vi "Get Descriptor_Mod.vi"(0 "VISA resource name":refnum<visa-resource-name>, 5 "Source (0: Channel 1)":u16(ring) items=["Channel 1", "Channel 2", "Channel 3", "Channel 4", "Memory 1", "Memory 2", "Memory 3", "Memory 4", "Function 1", "Function 2", "Function 3", "Function 4", "Function 5", "Function 6", "Function 7", "Function 8", "Other"], 7 "Custom Source ID":string, 11 "error in (no error)":errorcluster) -> (1 "First Valid Point":i32, 2 "Last Valid Point":i32, 3 "Horizontal interval":sgl, 4 "VISA resource name out":refnum<visa-resource-name>, 6 "Vertical gain":sgl, 8 "Horizontal Offset":dbl, 10 "Vertical offset":sgl, 12 "Number Of Data Points":i32, 13 "Nom_Bits":i16, 14 "Command type":i16, 15 "error out":errorcluster)   [LabVIEW 2022 SP3]
doc: "Get basic information about acquisition waveform from specified channel."
uses:
  <instrlib>/LeCroy Wave Series/LeCroy Wave Series.lvlib
panel:
  out "Trigger Time":T1
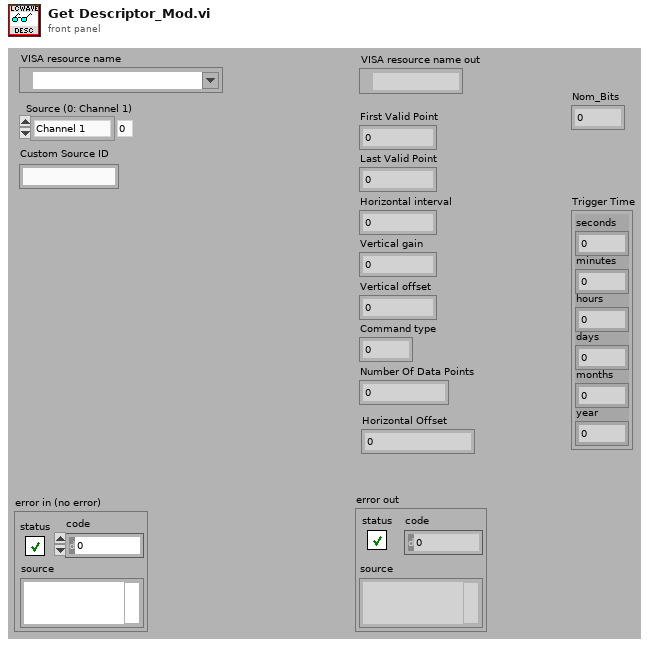
[diagram p1: front panel]
types:
  T1 = cluster{"seconds":dbl, "minutes":u8, "hours":u8, "days":u8, "months":u8, "year":u16}
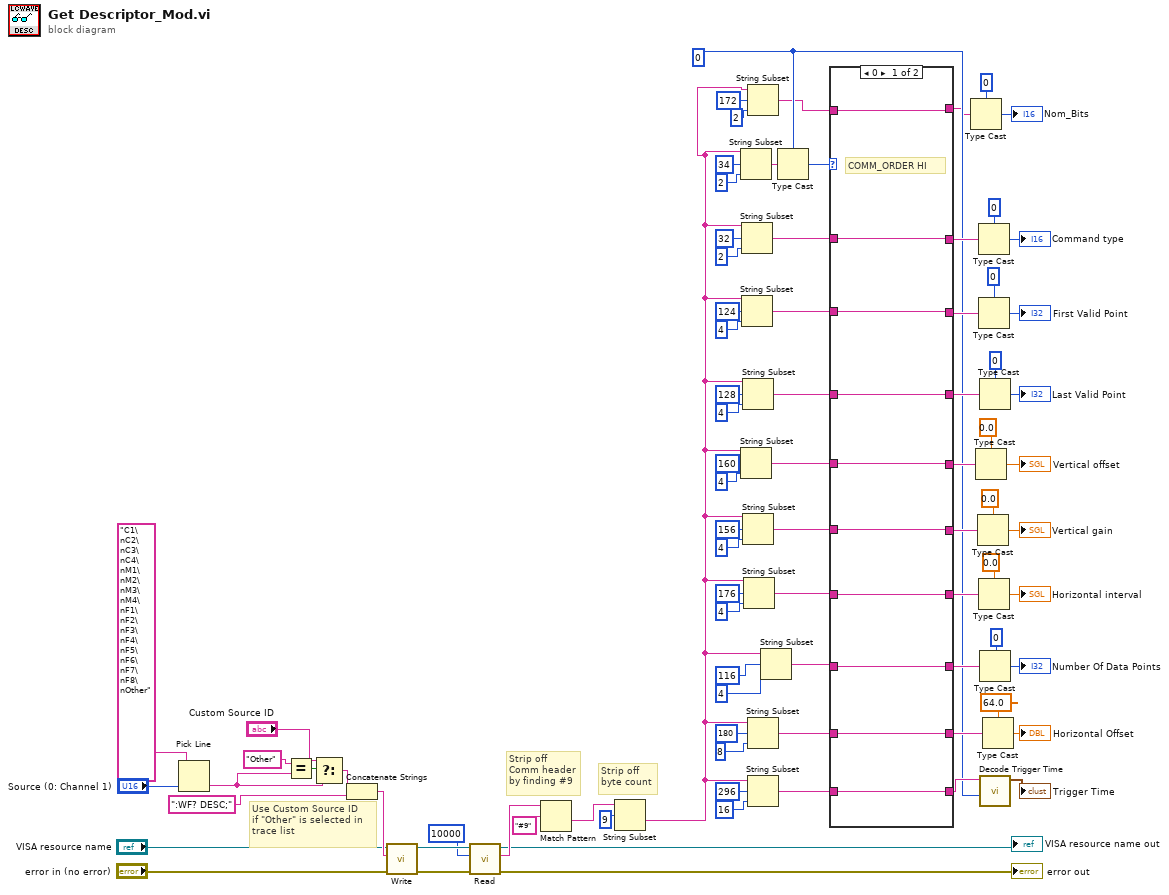
[diagram p0: block diagram]
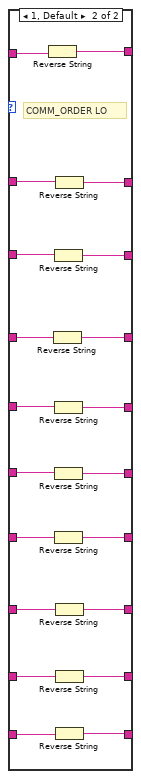
[diagram p2: hidden frame]
diagram:
  w8 = i16 0
  # "Use Custom Source ID\nif \"Other\" is selected in \ntrace list"
  # "Strip off byte count"
  # "Strip off\nComm header\nby finding #9"
  n1 = Pick Line(multi-line string="C1\nC2\nC3\nC4\nM1\nM2\nM3\nM4\nF1\nF2\nF3\nF4\nF5\nF6\nF7\nF8\nOther", line index="Source (0: Channel 1)") -> (output string=w21:string)  [unwired: 1 in]
  n2 = Equal?(x="Other", y=w21) -> (x = y?=w23:bool)
  n3 = Select(t="Custom Source ID", s=w23, f=w21) -> (s? t:f=w20:string)
  n4 = Concatenate Strings(w20, ":WF? DESC;" ("write buffer")) -> (w30:string)
  n5 = call <instrlib>:"Write.vi"("error in (no error)"="error in (no error)", "Write Buffer"=w30, "VISA resource name"="VISA resource name") -> ("error out"=w36:errorcluster, "VISA resource name out"=w28:refnum<visa-resource-name>)  [unwired: 6 in, 1 out]
  n6 = call <instrlib>:"Read.vi"("error in (no error)"=w36, "Byte Count"=u32 10000, "VISA resource name"=w28) -> ("error out"=→"error out":errorcluster, "Read Buffer"=w26:string, "VISA resource name out"=→"VISA resource name out":refnum<visa-resource-name>)  [unwired: 5 in, 1 out]
  n7 = Match Pattern(string=w26, regular expression="#9") -> (after substring=w37:string)  [unwired: 1 in, 3 out]
  n8 = String Subset(string=w37, offset (0)=9 ("length (rest)")) -> (substring=w4:string)  [unwired: 1 in]
  n9 = String Subset(string=w4, offset (0)=34, length (rest)=2 ("length (rest)")) -> (substring=w65:string)
  n10 = String Subset(string=w4, offset (0)=160, length (rest)=4 ("length (rest)")) -> (substring=w80:string)
  n11 = String Subset(string=w4, offset (0)=32, length (rest)=2 ("length (rest)")) -> (substring=w55:string)
  n12 = String Subset(string=w4, offset (0)=124, length (rest)=4 ("length (rest)")) -> (substring=w61:string)
  n13 = String Subset(string=w4, offset (0)=128, length (rest)=4 ("length (rest)")) -> (substring=w43:string)
  n14 = String Subset(string=w4, offset (0)=156, length (rest)=4 ("length (rest)")) -> (substring=w74:string)
  n15 = String Subset(string=w4, offset (0)=176, length (rest)=4 ("length (rest)")) -> (substring=w69:string)
  n16 = String Subset(string=w4, offset (0)=172, length (rest)=2 ("length (rest)")) -> (substring=w5:string)
  n17 = String Subset(string=w4, offset (0)=180, length (rest)=8 ("length")) -> (substring=w17:string)
  n18 = String Subset(string=w4, offset (0)=296, length (rest)=16 ("length (rest)")) -> (substring=w11:string)
  n19 = String Subset(string=w4, offset (0)=116, length (rest)=4 ("length (rest)")) -> (substring=w51:string)
  n20 = Type Cast(type=w8, x=w65) -> (*(type *) &x=w64:i16)
  n21 = case shown="0" w64 {
    tunnel: [w95 w115] -> w81
    tunnel: w80 -> [w95 w114]
    tunnel: [w94 w113] -> w75
    tunnel: w74 -> [w94 w112]
    tunnel: [w93 w111] -> w70
    tunnel: w69 -> [w93 w110]
    tunnel: w61 -> [w92 w109]
    tunnel: [w92 w108] -> w58
    tunnel: w55 -> [w91 w103]
    tunnel: [w91 w102] -> w53
    tunnel: [w90 w106] -> w50
    tunnel: w51 -> [w90 w107]
    tunnel: w43 -> [w89 w105]
    tunnel: [w89 w104] -> w42
    tunnel: w17 -> [w88 w101]
    tunnel: [w88 w100] -> w16
    tunnel: w11 -> [w87 w99]
    tunnel: [w87 w98] -> w10
    tunnel: w5 -> [w86 w97]
    tunnel: [w86 w96] -> w1
    frame 0 {
      # "COMM_ORDER HI"
    }
    frame 1, Default {
      # "COMM_ORDER LO"
      n22 = Reverse String(1:w97) -> (0:w96:string)
      n23 = Reverse String(1:w105) -> (0:w104:string)
      n24 = Reverse String(1:w109) -> (0:w108:string)
      n25 = Reverse String(1:w114) -> (0:w115:string)
      n26 = Reverse String(1:w112) -> (0:w113:string)
      n27 = Reverse String(1:w110) -> (0:w111:string)
      n28 = Reverse String(1:w103) -> (0:w102:string)
      n29 = Reverse String(1:w107) -> (0:w106:string)
      n30 = Reverse String(1:w101) -> (0:w100:string)
      n31 = Reverse String(1:w99) -> (0:w98:string)
    }
  }
  n32 = Type Cast(type=i16 0, x=w1) -> (*(type *) &x=→"Nom_Bits":i16)
  n33 = Type Cast(type=sgl 0.0, x=w81) -> (*(type *) &x=→"Vertical offset":sgl)
  n34 = Type Cast(type=sgl 0.0, x=w75) -> (*(type *) &x=→"Vertical gain":sgl)
  n35 = Type Cast(type=i16 0, x=w53) -> (*(type *) &x=→"Command type":i16)
  n36 = Type Cast(type=0, x=w58) -> (*(type *) &x=→"First Valid Point":i32)
  n37 = Type Cast(type=sgl 0.0, x=w70) -> (*(type *) &x=→"Horizontal interval":sgl)
  n38 = Type Cast(type=0, x=w42) -> (*(type *) &x=→"Last Valid Point":i32)
  n39 = Type Cast(type=0, x=w50) -> (*(type *) &x=→"Number Of Data Points":i32)
  n40 = call <instrlib>:"Decode Trigger Time.vi"("Comm_order"=w8, "Trigger_time string"=w10) -> ("Trigger Time"=→"Trigger Time":T1)  [unwired: 8 in]
  n41 = Type Cast(type=64.0, x=w16) -> (*(type *) &x=→"Horizontal Offset":dbl)
